vi "test-translation2d.vi"(8 "error in (no error)":errorcluster) -> (0 "error out":errorcluster, 3 "All PASSED":bool)   [LabVIEW 2019]
uses:
  <vilib>/Rock Robotics/WPI/ThirdParty/JAS_Junk/TrajLib/TypeDef/TRANSLATION2D.ctl
  <vilib>/Rock Robotics/WPI/ThirdParty/JAS_Junk/TrajLib/Rotation2d_GetAngleCosSin.vi
  <vilib>/Rock Robotics/WPI/ThirdParty/JAS_Junk/TrajLib/Util_CalcDist.vi
  <vilib>/Rock Robotics/WPI/ThirdParty/JAS_Junk/TrajLib/Trajectory_Library.lvlib
panel:
  out "T11 Nearest To":bool
  out "T10 X-7.79, Y=4.5":T1 {"Y" format="%14.3f"; "X" format="%14.3f"}
  out "T7 -- y -- 0":dbl
  out "T7 -- X -- 0":dbl
  out "T6 -- dist - 0":dbl
  out "T5 -- norm - 0":dbl
  out "T4 -- y -- 0":dbl
  out "T4 -- X -- 0":dbl
  out "T3 -- y -- 0":dbl
  out "T3 -- X -- 0":dbl
  out "T2 -- y -- 0":dbl
  out "T2 -- X -- 0":dbl
  out "T9 - False":bool
  out "T8 - True":bool
  out "T1 -- y -- 0":dbl
  out "T1 -- X -- 0":dbl
  out "T0 -- y -- 0":dbl
  out "T0 -- X -- 0":dbl
  # "Translation2D Test"
  # "Didn't implement divide"
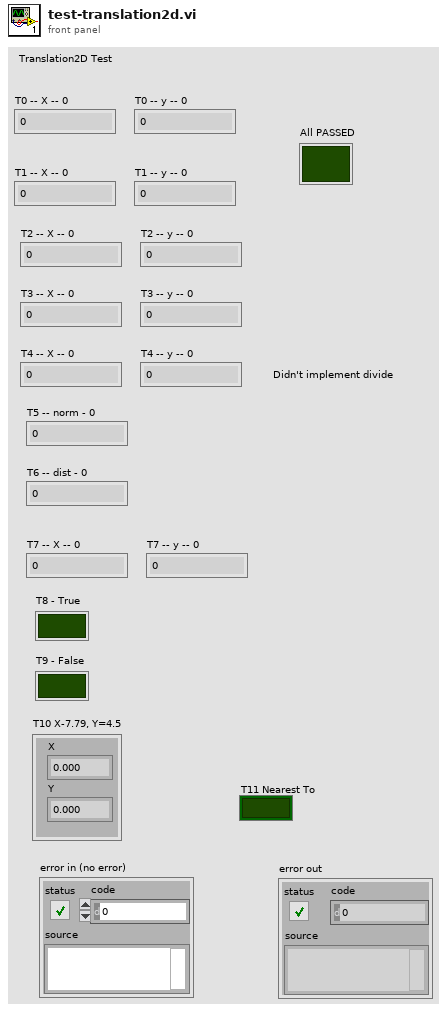
[diagram p1: front panel]
types:
  T1 = typedef "Trajectory_Library.lvlib/TRANSLATION2D.ctl" = cluster{"X":dbl, "Y":dbl}
  T2 = typedef "Trajectory_Library.lvlib/ROTATION2D.ctl" = cluster{"VALUE":dbl, "COS":dbl, "SIN":dbl}
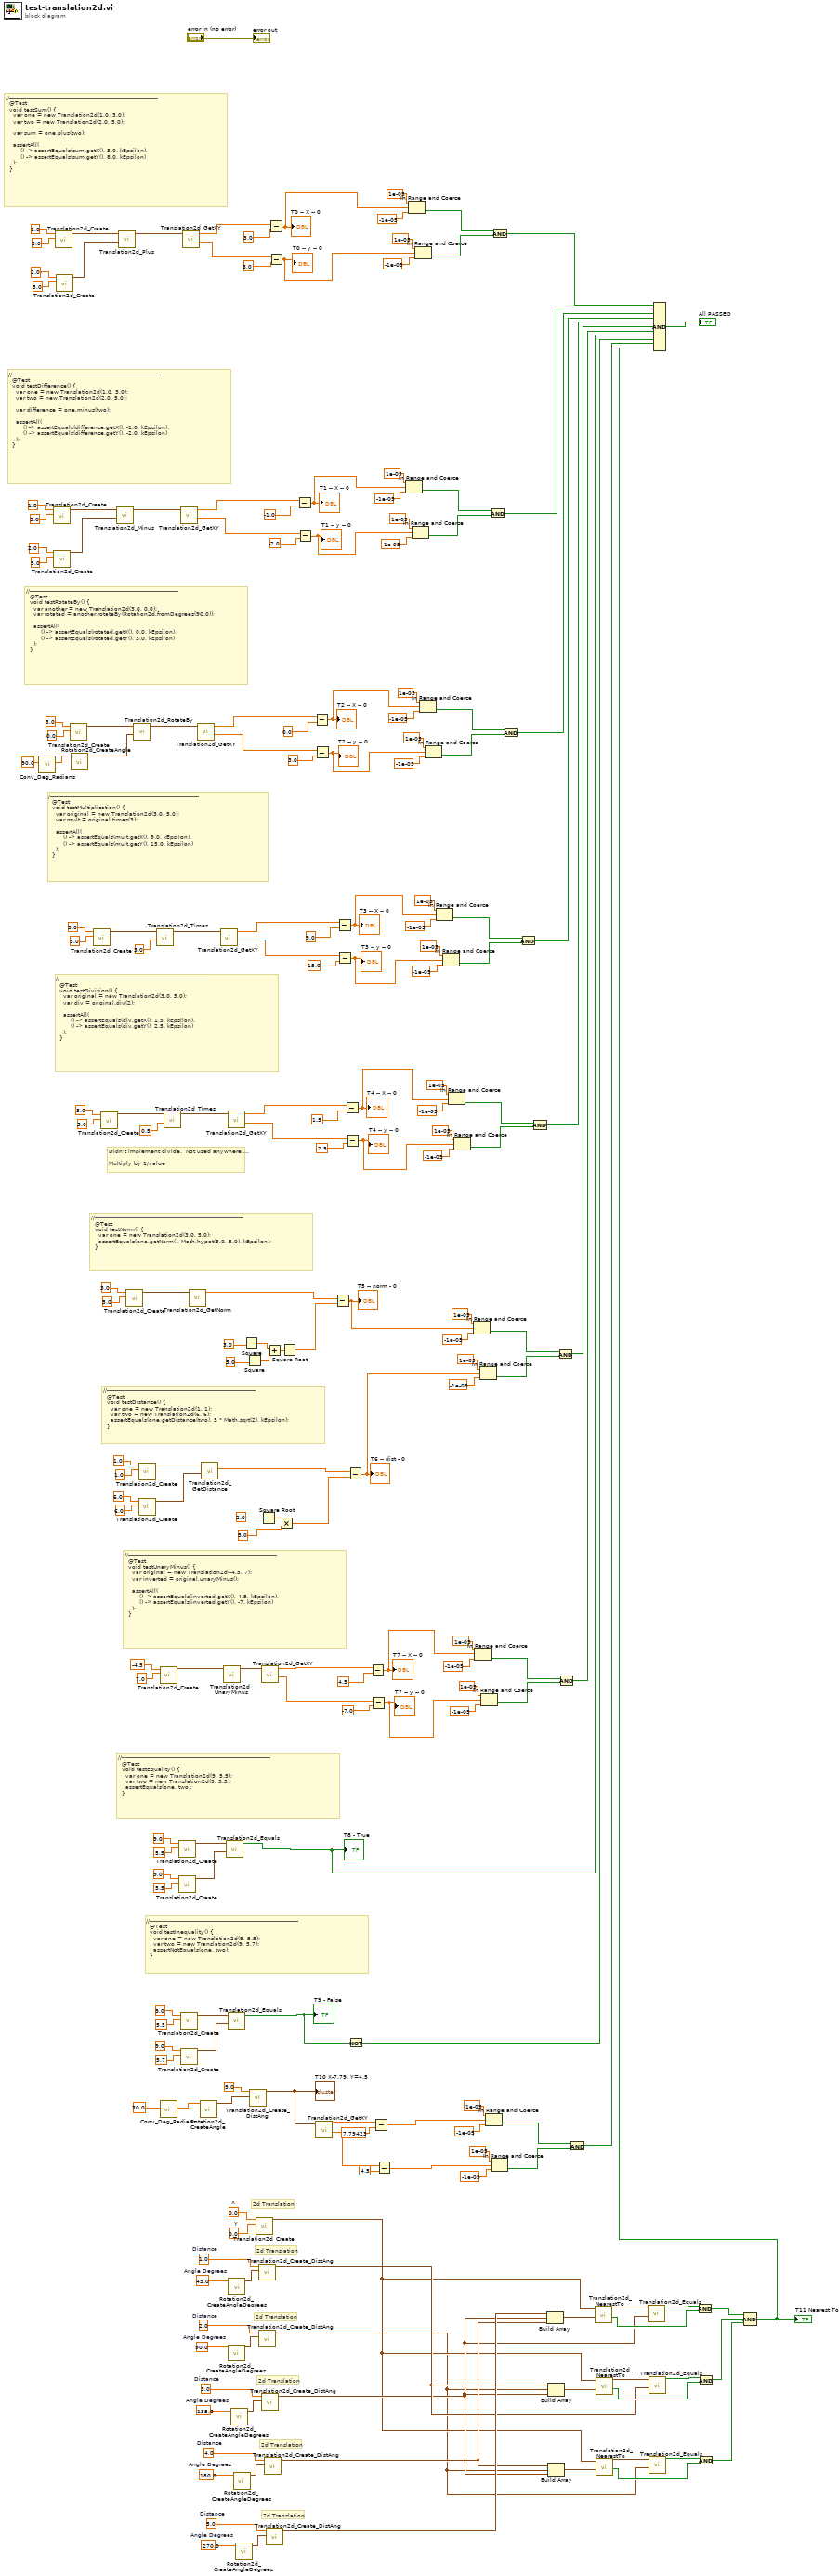
[diagram p0: block diagram]
diagram:
  w22 = 0.0  # X
  w21 = 0.0  # Y
  w25 = 5.0  # Distance
  w27 = 270.0  # Angle Degrees
  w28 = 4.0  # Distance
  w30 = 180.0  # Angle Degrees
  w31 = 3.0  # Distance
  w33 = 135.0  # Angle Degrees
  w34 = 2.0  # Distance
  w36 = 90.0  # Angle Degrees
  w37 = 1.0  # Distance
  w39 = 45.0  # Angle Degrees
  # "2d Translation"
  # "2d Translation"
  # "2d Translation"
  # "2d Translation"
  # "2d Translation"
  # "2d Translation"
  # "//--------------------------------------------------------------------------------\n  @Test\n  void testInequality() {\n    var one = new Translation2d(9, 5.5);\n    var two = new Translation2d(9, 5.7);\n    assertNotEquals(one, two);\n  }"
  # "//--------------------------------------------------------------------------------\n  @Test\n  void testUnaryMinus() {\n    var original = new Translation2d(-4.5, 7);\n    var inverted = original.unaryMinus();\n\n    assertAll(\n        () -> assertEquals(inverted.getX(), 4.5, kEpsilon),\n        () -> assertEquals(inverted.getY(), -7, kEpsilon)\n    );\n  }"
  # "//--------------------------------------------------------------------------------\n  @Test\n  void testDistance() {\n    var one = new Translation2d(1, 1);\n    var two = new Translation2d(6, 6);\n    assertEquals(one.getDistance(two), 5 * Math.sqrt(2), kEpsilon);\n  }"
  # "//--------------------------------------------------------------------------------\n  @Test\n  void testNorm() {\n    var one = new Translation2d(3.0, 5.0);\n    assertEquals(one.getNorm(), Math.hypot(3.0, 5.0), kEpsilon);\n  }"
  # "Didn't implement divide.  Not used anywhere....\n\nMultiply by 1/value"
  # "//--------------------------------------------------------------------------------\n  @Test\n  void testDivision() {\n    var original = new Translation2d(3.0, 5.0);\n    var div = original.div(2);\n\n    assertAll(\n        () -> assertEquals(div.getX(), 1.5, kEpsilon),\n        () -> assertEquals(div.getY(), 2.5, kEpsilon)\n    );\n  }"
  # "/--------------------------------------------------------------------------------\n  @Test\n  void testMultiplication() {\n    var original = new Translation2d(3.0, 5.0);\n    var mult = original.times(3);\n\n    assertAll(\n        () -> assertEquals(mult.getX(), 9.0, kEpsilon),\n        () -> assertEquals(mult.getY(), 15.0, kEpsilon)\n    );\n  }"
  # "//--------------------------------------------------------------------------------\n  @Test\n  void testRotateBy() {\n    var another = new Translation2d(3.0, 0.0);\n    var rotated = another.rotateBy(Rotation2d.fromDegrees(90.0));\n\n    assertAll(\n        () -> assertEquals(rotated.getX(), 0.0, kEpsilon),\n        () -> assertEquals(rotated.getY(), 3.0, kEpsilon)\n    );\n  }"
  # "//--------------------------------------------------------------------------------\n  @Test\n  void testEquality() {\n    var one = new Translation2d(9, 5.5);\n    var two = new Translation2d(9, 5.5);\n    assertEquals(one, two);\n  }"
  # "//--------------------------------------------------------------------------------\n  @Test\n  void testDifference() {\n    var one = new Translation2d(1.0, 3.0);\n    var two = new Translation2d(2.0, 5.0);\n\n    var difference = one.minus(two);\n\n    assertAll(\n        () -> assertEquals(difference.getX(), -1.0, kEpsilon),\n        () -> assertEquals(difference.getY(), -2.0, kEpsilon)\n    );\n  }"
  # "//--------------------------------------------------------------------------------\n  @Test\n  void testSum() {\n    var one = new Translation2d(1.0, 3.0);\n    var two = new Translation2d(2.0, 5.0);\n\n    var sum = one.plus(two);\n\n    assertAll(\n        () -> assertEquals(sum.getX(), 3.0, kEpsilon),\n        () -> assertEquals(sum.getY(), 8.0, kEpsilon)\n    );\n  }"
  n1 = call <vilib>:"Conv_Deg_Radians.vi"("Degress"=90.0) -> ("Radians"=w187:dbl)  [unwired: 10 in]
  n2 = call <vilib>:"Translation2d_Create.vi"("Y"=3.0, "X"=1.0) -> ("TRANSLATION"=w201:T1)  [unwired: 9 in]
  n3 = call <vilib>:"Translation2d_Create.vi"("Y"=5.0, "X"=2.0) -> ("TRANSLATION"=w200:T1)  [unwired: 9 in]
  n4 = call <vilib>:"Translation2d_Create.vi"("Y"=3.0, "X"=1.0) -> ("TRANSLATION"=w210:T1)  [unwired: 9 in]
  n5 = call <vilib>:"Translation2d_Create.vi"("Y"=5.0, "X"=2.0) -> ("TRANSLATION"=w209:T1)  [unwired: 9 in]
  n6 = call <vilib>:"Translation2d_Create.vi"("Y"=0.0, "X"=3.0) -> ("TRANSLATION"=w192:T1)  [unwired: 9 in]
  n7 = call <vilib>:"Rotation2d_CreateAngle.vi"("Angle"=w187) -> ("ROTATION"=w185:T2)  [unwired: 10 in]
  n8 = call <vilib>:"Translation2d_Create.vi"("Y"=5.0, "X"=3.0) -> ("TRANSLATION"=w181:T1)  [unwired: 9 in]
  n9 = call <vilib>:"Translation2d_Create.vi"("Y"=5.0, "X"=3.0) -> ("TRANSLATION"=w172:T1)  [unwired: 9 in]
  n10 = call <vilib>:"Translation2d_Minus.vi"("other Translation"=w200, "In Translation"=w201) -> ("Out Translation"=w199:T1)  [unwired: 9 in]
  n11 = call <vilib>:"Translation2d_Plus.vi"("other Translation"=w209, "In Translation"=w210) -> ("Out Translation"=w208:T1)  [unwired: 9 in]
  n12 = call <vilib>:"Translation2d_Create.vi"("Y"=5.0, "X"=3.0) -> ("TRANSLATION"=w164:T1)  [unwired: 9 in]
  n13 = call <vilib>:"Translation2d_RotateBy.vi"("other Rotation"=w185, "In Translation"=w192) -> ("Out Translation"=w191:T1)  [unwired: 9 in]
  n14 = call <vilib>:"Translation2d_Create.vi"("Y"=1.0, "X"=1.0) -> ("TRANSLATION"=w154:T1)  [unwired: 9 in]
  n15 = call <vilib>:"Translation2d_Create.vi"("Y"=6.0, "X"=6.0) -> ("TRANSLATION"=w150:T1)  [unwired: 9 in]
  n16 = call <vilib>:"Translation2d_Times.vi"("Scalar"=3.0, "In Translation"=w181) -> ("Out Translation"=w180:T1)  [unwired: 9 in]
  n17 = call <vilib>:"Translation2d_Create.vi"("Y"=7.0, "X"=-4.5) -> ("TRANSLATION"=w143:T1)  [unwired: 9 in]
  n18 = call <vilib>:"Conv_Deg_Radians.vi"("Degress"=30.0 ("Y")) -> ("Radians"=w123:dbl)  [unwired: 10 in]
  n19 = call <vilib>:"Translation2d_Times.vi"("Scalar"=0.5, "In Translation"=w172) -> ("Out Translation"=w171:T1)  [unwired: 9 in]
  n20 = call <vilib>:"Translation2d_Create.vi"("Y"=5.5, "X"=9.0) -> ("TRANSLATION"=w133:T1)  [unwired: 9 in]
  n21 = call <vilib>:"Translation2d_Create.vi"("Y"=5.5, "X"=9.0) -> ("TRANSLATION"=w132:T1)  [unwired: 9 in]
  n22 = call <vilib>:"Translation2d_GetXY.vi"("In Translation"=w199) -> ("Y"=w197:dbl, "X"=w198:dbl)  [unwired: 9 in]
  n23 = call <vilib>:"Translation2d_Create.vi"("Y"=5.5, "X"=9.0) -> ("TRANSLATION"=w127:T1)  [unwired: 9 in]
  n24 = call <vilib>:"Translation2d_Create.vi"("Y"=5.7, "X"=9.0) -> ("TRANSLATION"=w126:T1)  [unwired: 9 in]
  n25 = call <vilib>:"Translation2d_GetXY.vi"("In Translation"=w208) -> ("Y"=w212:dbl, "X"=w213:dbl)  [unwired: 9 in]
  n26 = call <vilib>:"Translation2d_GetNorm.vi"("In Translation"=w164) -> ("Norm"=w158:dbl)  [unwired: 10 in]
  n27 = call <vilib>:"Translation2d_GetXY.vi"("In Translation"=w191) -> ("Y"=w189:dbl, "X"=w190:dbl)  [unwired: 9 in]
  n28 = call <vilib>:"Rotation2d_CreateAngle.vi"("Angle"=w123) -> ("ROTATION"=w124:T2)  [unwired: 10 in]
  n29 = call <vilib>:"Translation2d_GetDistance.vi"("other Translation"=w150, "In Translation"=w154) -> ("Distance"=w153:dbl)  [unwired: 9 in]
  n30 = call <vilib>:"Translation2d_GetXY.vi"("In Translation"=w180) -> ("Y"=w178:dbl, "X"=w179:dbl)  [unwired: 9 in]
  n31 = call <vilib>:"Translation2d_UnaryMinus.vi"("In Translation"=w143) -> ("Out Translation"=w140:T1)  [unwired: 10 in]
  n32 = call <vilib>:"Translation2d_Equals.vi"("other Translation"=w132, "In Translation"=w133) -> ("Equals"=w57:bool)  [unwired: 9 in]
  "T8 - True" <- w57
  n33 = call <vilib>:"Translation2d_GetXY.vi"("In Translation"=w171) -> ("Y"=w169:dbl, "X"=w170:dbl)  [unwired: 9 in]
  n34 = call <vilib>:"Translation2d_Equals.vi"("other Translation"=w126, "In Translation"=w127) -> ("Equals"=w56:bool)  [unwired: 9 in]
  "T9 - False" <- w56
  n35 = call <vilib>:"Rotation2d_CreateAngleDegrees.vi"("Angle_Degrees"=w36) -> ("ROTATION"=w35:T2)  [unwired: 10 in]
  n36 = call <vilib>:"Rotation2d_CreateAngleDegrees.vi"("Angle_Degrees"=w39) -> ("ROTATION"=w38:T2)  [unwired: 10 in]
  n37 = call <vilib>:"Rotation2d_CreateAngleDegrees.vi"("Angle_Degrees"=w33) -> ("ROTATION"=w32:T2)  [unwired: 10 in]
  n38 = call <vilib>:"Rotation2d_CreateAngleDegrees.vi"("Angle_Degrees"=w30) -> ("ROTATION"=w29:T2)  [unwired: 10 in]
  n39 = call <vilib>:"Rotation2d_CreateAngleDegrees.vi"("Angle_Degrees"=w27) -> ("ROTATION"=w26:T2)  [unwired: 10 in]
  n40 = Square(x=3.0 ("X")) -> (x^2=w160:dbl)
  n41 = Square(x=5.0 ("X")) -> (x^2=w159:dbl)
  n42 = call <vilib>:"Translation2d_Create_DistAng.vi"("Angle"=w124, "Dist"=9.0 ("X")) -> ("TRANSLATION"=w48:T1)  [unwired: 9 in]
  "T10 X-7.79, Y=4.5" <- w48
  n43 = call <vilib>:"Translation2d_Create.vi"("Y"=w21, "X"=w22) -> ("TRANSLATION"=w5:T1)  [unwired: 9 in]
  n44 = call <vilib>:"Translation2d_Create_DistAng.vi"("Angle"=w35, "Dist"=w34) -> ("TRANSLATION"=w4:T1)  [unwired: 9 in]
  n45 = call <vilib>:"Translation2d_Create_DistAng.vi"("Angle"=w38, "Dist"=w37) -> ("TRANSLATION"=w12:T1)  [unwired: 9 in]
  n46 = Square Root(x=2.0 ("X")) -> (sqrt(x)=w148:dbl)
  n47 = call <vilib>:"Translation2d_GetXY.vi"("In Translation"=w140) -> ("Y"=w138:dbl, "X"=w139:dbl)  [unwired: 9 in]
  n48 = call <vilib>:"Translation2d_Create_DistAng.vi"("Angle"=w32, "Dist"=w31) -> ("TRANSLATION"=w6:T1)  [unwired: 9 in]
  n49 = call <vilib>:"Translation2d_Create_DistAng.vi"("Angle"=w29, "Dist"=w28) -> ("TRANSLATION"=w7:T1)  [unwired: 9 in]
  n50 = Add(x=w160, y=w159) -> (x+y=w161:dbl)
  n51 = call <vilib>:"Translation2d_Create_DistAng.vi"("Angle"=w26, "Dist"=w25) -> ("TRANSLATION"=w24:T1)  [unwired: 9 in]
  n52 = Subtract(x=w213, y=3.0) -> (x-y=w113:dbl)
  "T0 -- X -- 0" <- w113
  n53 = Subtract(x=w212, y=8.0) -> (x-y=w112:dbl)
  "T0 -- y -- 0" <- w112
  n54 = Multiply(x=w148, y=5.0 ("X")) -> (x*y=w146:dbl)
  n55 = Square Root(x=w161) -> (sqrt(x)=w157:dbl)
  n56 = Subtract(x=w198, y=-1.0 ("x")) -> (x-y=w105:dbl)
  "T1 -- X -- 0" <- w105
  n57 = Subtract(x=w197, y=-2.0) -> (x-y=w104:dbl)
  "T1 -- y -- 0" <- w104
  n58 = Subtract(x=w190, y=0.0 ("x")) -> (x-y=w96:dbl)
  "T2 -- X -- 0" <- w96
  n59 = Subtract(x=w189, y=3.0) -> (x-y=w95:dbl)
  "T2 -- y -- 0" <- w95
  n60 = call <vilib>:"Translation2d_GetXY.vi"("In Translation"=w48) -> ("Y"=w46:dbl, "X"=w47:dbl)  [unwired: 9 in]
  n61 = Subtract(x=w158, y=w157) -> (x-y=w69:dbl)
  "T5 -- norm - 0" <- w69
  n62 = Subtract(x=w179, y=9.0 ("x")) -> (x-y=w80:dbl)
  "T3 -- X -- 0" <- w80
  n63 = Subtract(x=w178, y=15.0) -> (x-y=w79:dbl)
  "T3 -- y -- 0" <- w79
  n64 = Subtract(x=w170, y=1.5 ("x")) -> (x-y=w78:dbl)
  "T4 -- X -- 0" <- w78
  n65 = Subtract(x=w169, y=2.5) -> (x-y=w77:dbl)
  "T4 -- y -- 0" <- w77
  n66 = Subtract(x=w153, y=w146) -> (x-y=w68:dbl)
  "T6 -- dist - 0" <- w68
  n67 = Not(x=w56) -> (.not. x?=w55:bool)
  n68 = Subtract(x=w139, y=4.5 ("x")) -> (x-y=w60:dbl)
  "T7 -- X -- 0" <- w60
  n69 = Subtract(x=w138, y=-7.0) -> (x-y=w59:dbl)
  "T7 -- y -- 0" <- w59
  n70 = Subtract(x=w47, y=7.79423) -> (x-y=w43:dbl)
  n71 = Subtract(x=w46, y=4.5) -> (x-y=w42:dbl)
  n72 = In Range and Coerce(upper limit=1e-05, x=w105, lower limit=-1e-05) -> (In Range?=w107:bool)  [unwired: 1 out]
  n73 = In Range and Coerce(upper limit=1e-05, x=w113, lower limit=-1e-05) -> (In Range?=w117:bool)  [unwired: 1 out]
  n74 = In Range and Coerce(upper limit=1e-05, x=w104, lower limit=-1e-05) -> (In Range?=w106:bool)  [unwired: 1 out]
  n75 = In Range and Coerce(upper limit=1e-05, x=w112, lower limit=-1e-05) -> (In Range?=w116:bool)  [unwired: 1 out]
  n76 = In Range and Coerce(upper limit=1e-05, x=w96, lower limit=-1e-05) -> (In Range?=w98:bool)  [unwired: 1 out]
  n77 = In Range and Coerce(upper limit=1e-05, x=w95, lower limit=-1e-05) -> (In Range?=w97:bool)  [unwired: 1 out]
  n78 = In Range and Coerce(upper limit=1e-05, x=w80, lower limit=-1e-05) -> (In Range?=w89:bool)  [unwired: 1 out]
  n79 = In Range and Coerce(upper limit=1e-05, x=w79, lower limit=-1e-05) -> (In Range?=w88:bool)  [unwired: 1 out]
  n80 = In Range and Coerce(upper limit=1e-05, x=w78, lower limit=-1e-05) -> (In Range?=w83:bool)  [unwired: 1 out]
  n81 = In Range and Coerce(upper limit=1e-05, x=w77, lower limit=-1e-05) -> (In Range?=w82:bool)  [unwired: 1 out]
  n82 = In Range and Coerce(upper limit=1e-05, x=w69, lower limit=-1e-05) -> (In Range?=w71:bool)  [unwired: 1 out]
  n83 = In Range and Coerce(upper limit=1e-05, x=w60, lower limit=-1e-05) -> (In Range?=w62:bool)  [unwired: 1 out]
  n84 = In Range and Coerce(upper limit=1e-05, x=w68, lower limit=-1e-05) -> (In Range?=w70:bool)  [unwired: 1 out]
  n85 = In Range and Coerce(upper limit=1e-05, x=w59, lower limit=-1e-05) -> (In Range?=w61:bool)  [unwired: 1 out]
  n86 = In Range and Coerce(upper limit=1e-05, x=w43, lower limit=-1e-05) -> (In Range?=w50:bool)  [unwired: 1 out]
  n87 = Compound Arithmetic op=AND(w107, w106) -> (w103:bool)
  n88 = In Range and Coerce(upper limit=1e-05, x=w42, lower limit=-1e-05) -> (In Range?=w49:bool)  [unwired: 1 out]
  n89 = Compound Arithmetic op=AND(w117, w116) -> (w115:bool)
  n90 = Compound Arithmetic op=AND(w98, w97) -> (w94:bool)
  n91 = Compound Arithmetic op=AND(w89, w88) -> (w81:bool)
  n92 = Compound Arithmetic op=AND(w83, w82) -> (w76:bool)
  n93 = Build Array(w24, w6, w7) -> (w23:T1[])
  n94 = Build Array(w12, w4, w6) -> (w16:T1[])
  n95 = Build Array(w7, w4, w6) -> (w11:T1[])
  n96 = Compound Arithmetic op=AND(w71, w70) -> (w67:bool)
  n97 = Compound Arithmetic op=AND(w62, w61) -> (w58:bool)
  n98 = Compound Arithmetic op=AND(w50, w49) -> (w41:bool)
  n99 = call <vilib>:"Translation2d_NearestTo.vi"("Other Translations"=w23, "In Translation"=w5) -> ("Found"=w19:bool, "Nearest Translation"=w20:T1)  [unwired: 8 in]
  n100 = call <vilib>:"Translation2d_NearestTo.vi"("Other Translations"=w16, "In Translation"=w5) -> ("Found"=w14:bool, "Nearest Translation"=w15:T1)  [unwired: 8 in]
  n101 = call <vilib>:"Translation2d_NearestTo.vi"("Other Translations"=w11, "In Translation"=w5) -> ("Found"=w9:bool, "Nearest Translation"=w10:T1)  [unwired: 8 in]
  n102 = call <vilib>:"Translation2d_Equals.vi"("other Translation"=w6, "In Translation"=w20) -> ("Equals"=w18:bool)  [unwired: 9 in]
  n103 = call <vilib>:"Translation2d_Equals.vi"("other Translation"=w12, "In Translation"=w15) -> ("Equals"=w13:bool)  [unwired: 9 in]
  n104 = call <vilib>:"Translation2d_Equals.vi"("other Translation"=w4, "In Translation"=w10) -> ("Equals"=w8:bool)  [unwired: 9 in]
  n105 = And(x=w18, y=w19) -> (x .and. y?=w17:bool)
  n106 = And(x=w13, y=w14) -> (x .and. y?=w3:bool)
  n107 = And(x=w8, y=w9) -> (x .and. y?=w2:bool)
  n108 = Compound Arithmetic op=AND(w17, w3, w2) -> (w1:bool)
  "T11 Nearest To" <- w1
  n109 = Compound Arithmetic op=AND(w115, w103, w94, w81, w76, w67, w58, w57, w55, w41, w1) -> (→"All PASSED":bool)
  "error out" <- "error in (no error)"
